vi "Fully Custom Collection Page.vi"(8 "error in (no error)":errorcluster, 11 "Node Ptr":T1 format="%.0x") -> (0 "error out":errorcluster)   [LabVIEW 2011, in "Engine Sim System Explorer.lvlib"]
uses:
  Engine Sim System Explorer.lvlib
  <vilib>/NI Veristand/Custom Device API/Custom Device API.lvlib
  Shared/Engine Simulation Global.vi
  Engine Simulation Shared.lvlib
  <vilib>/NI Veristand/Custom Device API/Set Item Property (U16).vi
  <vilib>/NI Veristand/Custom Device API/Get Item Property (U16).vi
  <vilib>/NI Veristand/Custom Device API/Custom Device Item Ref.ctl
panel:
  in  "Number of Teeth":u16
  in  "SHDocVw.IWebBrowser2":refnum<k7>(container)
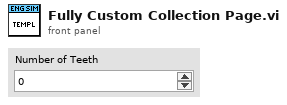
[diagram p1: front panel]
types:
  T1 = typedef "Custom Device API.lvlib/Custom Device Item Ref.ctl" = u64
  T2 = typedef "Custom Device API.lvlib/Custom Device Commands.ctl" = enum16{"Default", "Item renamed", "Shutdown", "Dynamic button pressed"}
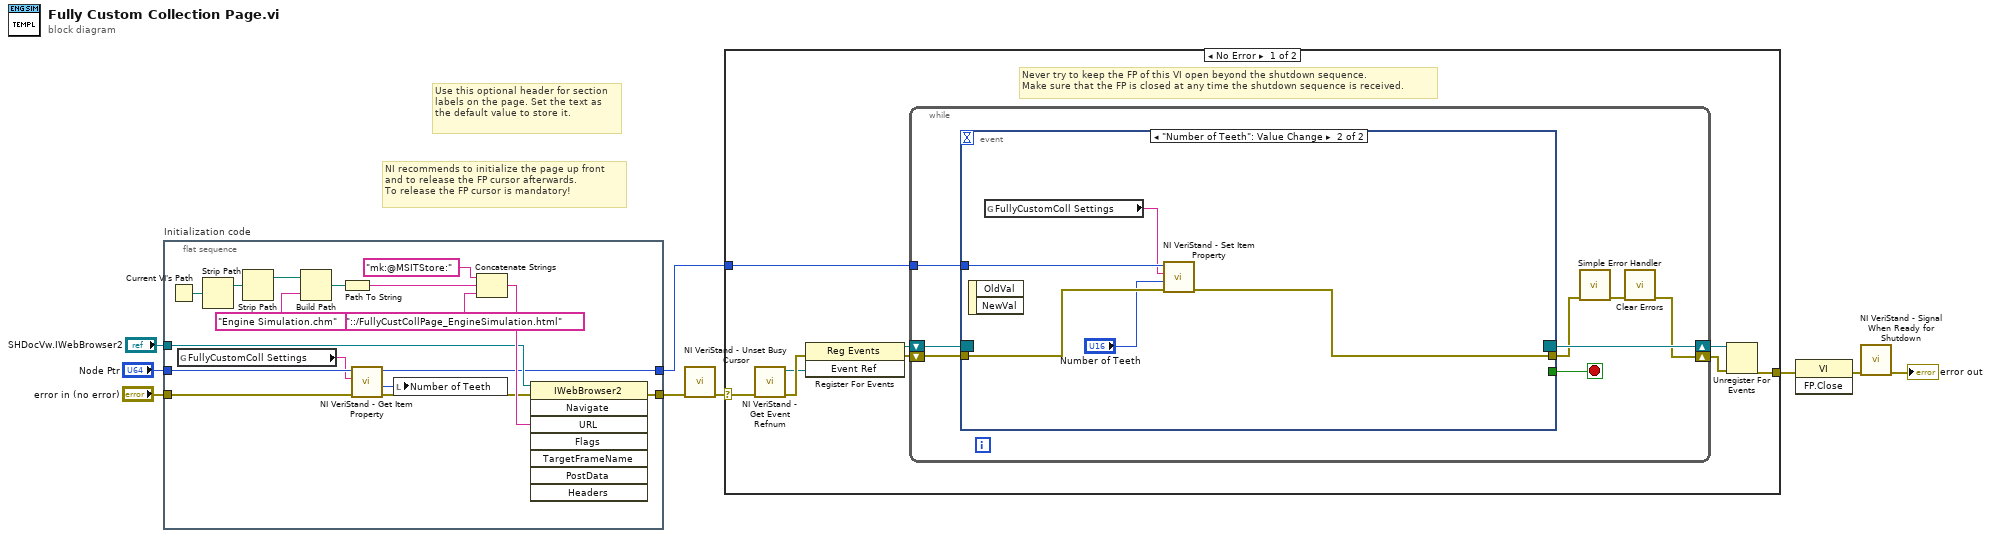
[diagram p0: block diagram]
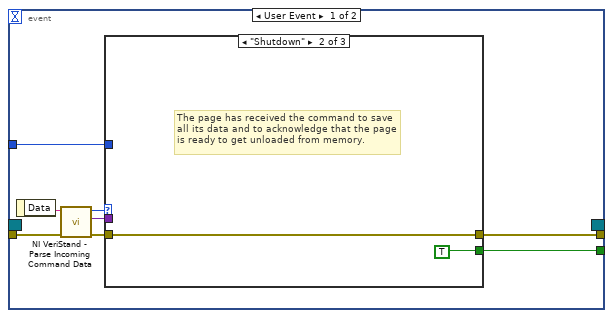
[diagram p2: hidden frame]
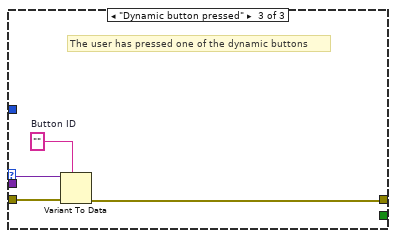
[diagram p4: hidden frame]
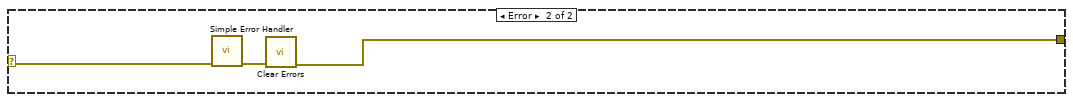
[diagram p5: hidden frame]
diagram:
  # "Use this optional header for section labels on the page. Set the text as the default value to store it."
  # "NI recommends to initialize the page up front\nand to release the FP cursor afterwards.\nTo release the FP cursor is mandatory!"
  n1 = flat-sequence "Initialization code" {
    tunnel: "error in (no error)" -> [w15]
    tunnel: "Node Ptr" -> [w14]
    tunnel: [w18] -> w5
    tunnel: [w13] -> w2
    tunnel: "SHDocVw.IWebBrowser2" -> [w16]
    frame #0 {
      n2 = Current VI's Path() -> (path=w20:path)
      n3 = global read "Engine Simulation Global.vi" "FullyCustomColl Settings"() -> (w10:string)
      n4 = Strip Path(path=w20) -> (stripped path=w21:path)  [unwired: 1 out]
      n5 = Strip Path(path=w21) -> (stripped path=w26:path)  [unwired: 1 out]
      n6 = Build Path(base path=w26, name or relative path="Engine Simulation.chm") -> (appended path=w24:path)
      n7 = Path To String(path=w24) -> (string=w23:string)
      n8 = call-poly <vilib>:"NI VeriStand - Get Item Property.vi"("error in (no error)"=w15, "Property Name"=w10, "Item Ref in"=w14) -> ("error out"=w12:errorcluster, "Value"=w11:u16, "Item Ref out"=w13:T1)  [unwired: 5 in, 1 out]
      n9 = local write "Number of Teeth"(w11) -> ()
      n10 = Concatenate Strings("mk:@MSITStore:" ("string"), w23, "::/FullyCustCollPage_EngineSimulation.html" ("name or relative path")) -> (w17:string)
      n11 = invoke class="IWebBrowser2" method="Navigate"(reference=w16, error in=w12, "URL"=w17) -> (error out=w18:errorcluster)  [unwired: 5 in, 7 out]
    }
  }
  n12 = call <vilib>:"NI VeriStand - Unset Busy Cursor.vi"("error in (no error)"=w5) -> ("error out"=w4:errorcluster)  [unwired: 10 out]
  n13 = case shown="No Error" w4 {
    selector: w4 -> [w27 w66]
    tunnel: [w32 w64] -> w9
    tunnel: w2 -> [w28 _]
    frame No Error {
      # "Never try to keep the FP of this VI open beyond the shutdown sequence.\nMake sure that the FP is closed at any time the shutdown sequence is received."
      n14 = call <vilib>:"NI VeriStand - Get Event Refnum.vi"("error in (no error)"=w27) -> ("error out"=w35:errorcluster, "Event Ref"=w31:refnum<user-event>)  [unwired: 9 out]
      n15 = register-events(error in=w35, w31) -> (reference out=w29:refnum<event-registration>, error out=w30:errorcluster)  [unwired: 1 in]
      n16 = while {
        tunnel: w28 -> [w39]
        shift-right: [w36] -> w33
        shift-left: w30 -> [w42]
        shift-right: [w43] -> w34
        shift-left: w29 -> [w41]
        stop <- w40 stop-if-true
        n17 = event shown="[1] \"Number of Teeth\": Value Change" {
          selector: w41 -> [_ _]
          dyn-events: [_ _] -> w43
          timeout: _ -> [_ _]
          tunnel: w42 -> [w51 w62]
          tunnel: [w47 _] -> w40
          tunnel: [w46 w59] -> w38
          tunnel: w39 -> [w45 w63]
          event User Event {
            n18 = event-data() -> ("Data"=w50:string)  [unwired: 1 out]
            n19 = call <vilib>:"NI VeriStand - Parse Incoming Command Data.vi"("error in (no error)"=w51, "Incoming data"=w50) -> ("error out"=w49:errorcluster, "Outgoing data"=w44:variant, "Action"=w48:T2)  [unwired: 7 out]
            n20 = case shown="\"Shutdown\"" w48 {
              tunnel: w49 -> [w52 w53 w58]
              tunnel: [_ TRUE _] -> w47
              tunnel: [w52 w53 w55] -> w46
              tunnel: w45 -> [_ _ _]
              tunnel: w44 -> [_ _ w57]
              frame "Default", Default {
              }
              frame "Shutdown" {
                # "The page has received the command to save all its data and to acknowledge that the page is ready to get unloaded from memory."
              }
              frame "Dynamic button pressed" {
                w56 = ""  # Button ID
                # "The user has pressed one of the dynamic buttons"
                n21 = Variant To Data(error in=w58, type=w56, Variant=w57) -> (error out=w55:errorcluster)  [unwired: 1 out]
              }
            }
          }
          event "Number of Teeth": Value Change {
            n22 = event-data() -> ()  [unwired: 3 out]
            n23 = global read "Engine Simulation Global.vi" "FullyCustomColl Settings"() -> (w61:string)
            n24 = call-poly <vilib>:"NI VeriStand - Set Item Property.vi"("error in (no error)"=w62, "Value"="Number of Teeth", "Property Name"=w61, "Item Ref in"=w63) -> ("error out"=w59:errorcluster)  [unwired: 5 in, 2 out]
          }
        }
        n25 = call <vilib>:"Simple Error Handler.vi"("error in (no error)"=w38) -> ("error out"=w37:errorcluster)  [unwired: 1 in, 7 out]
        n26 = call <vilib>:"Clear Errors.vi"("error in (no error)"=w37) -> ("error out"=w36:errorcluster)  [unwired: 6 out]
      }
      n27 = Unregister For Events(event registration refnum=w34, error in=w33) -> (error out=w32:errorcluster)
    }
    frame Error {
      n28 = call <vilib>:"Simple Error Handler.vi"("error in (no error)"=w66) -> ("error out"=w65:errorcluster)  [unwired: 1 in, 7 out]
      n29 = call <vilib>:"Clear Errors.vi"("error in (no error)"=w65) -> ("error out"=w64:errorcluster)  [unwired: 6 out]
    }
  }
  n30 = invoke class="VI" method="FP.Close"(error in=w9) -> (error out=w8:errorcluster)  [unwired: 2 in, 2 out]
  n31 = call <vilib>:"NI VeriStand - Signal When Ready for Shutdown.vi"("error in (no error)"=w8) -> ("error out"=→"error out":errorcluster)  [unwired: 10 out]
